vi "Get Rx and Tx Status Channels for Message.vi"(8 "error in":errorcluster, 11 "message refs":T1[](array[typedef]) format="%.0x") -> (0 "error out":errorcluster, 1 "Rx status channels":T1[](array[typedef]) format="%.0x", 2 "Tx status channels":T1[](array[typedef]) format="%.0x", 3 "message refs":T1[](array[typedef]) format="%.0x")   [LabVIEW 2023, in "Ballard MIL-STD-1553 Scripting.lvlib"]
uses:
  Ballard MIL-STD-1553 Scripting.lvlib
  <vilib>/NI VeriStand/Custom Device API/Custom Device Item Ref.ctl
  Shared/Direction.ctl
  Constants.vi
  <vilib>/NI VeriStand/Custom Device API/Custom Device API.lvlib
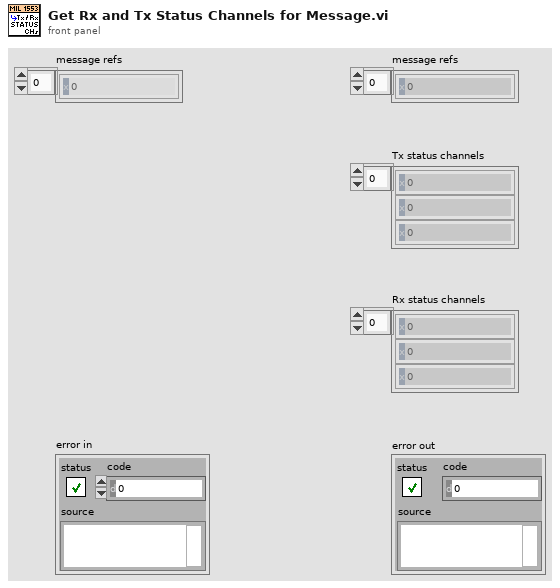
[diagram p1: front panel]
types:
  T1 = typedef "Custom Device API.lvlib/Custom Device Item Ref.ctl" = u64
  T2 = typedef "Direction.ctl" = enum16{"Rx", "Tx"}
  T3 = typedef "Message Type.ctl" = string
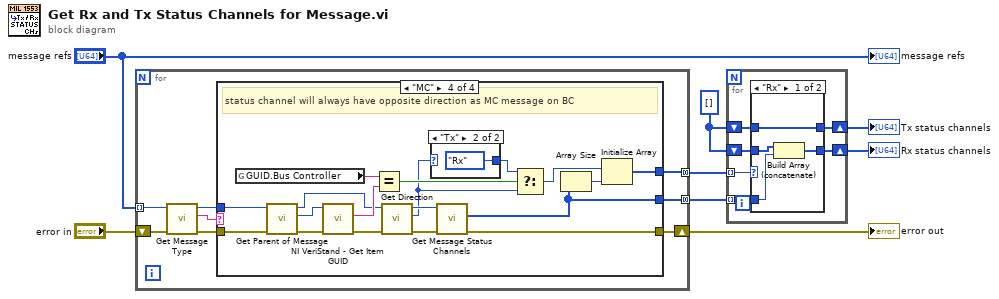
[diagram p0: block diagram]
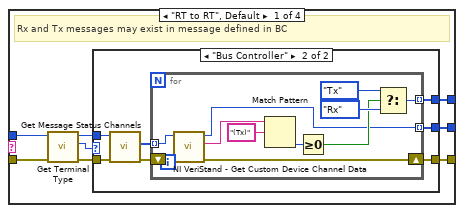
[diagram p2: hidden frame]
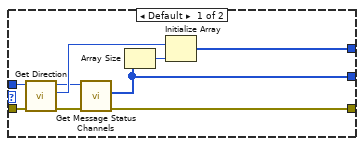
[diagram p3: hidden frame]
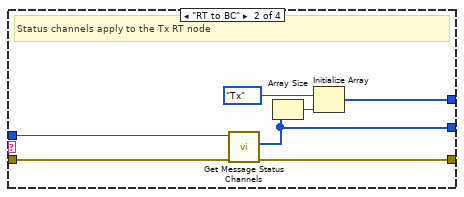
[diagram p4: hidden frame]
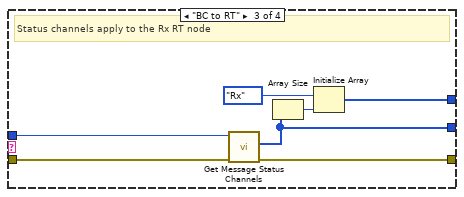
[diagram p5: hidden frame]
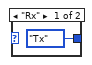
[diagram p6: hidden frame]
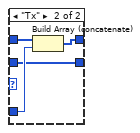
[diagram p7: hidden frame]
diagram:
  w6 = T1[] [] ("Rx status channels")
  n1 = for {
    tunnel: [w10] -> w3 mode=concatenating
    shift-right: [w11] -> w1
    shift-left: "error in" -> [w15]
    tunnel: "message refs" -> [w16] mode=indexing
    tunnel: [w9] -> w2 mode=concatenating
    n2 = call "Get Message Type.vi"("error in"=w15, "message in"=w16) -> ("error out"=w13:errorcluster, "message type"=w14:T3, "message out"=w12:T1)  [unwired: 6 in, 1 out]
    n3 = case shown="\"MC\"" w14 {
      tunnel: w13 -> [w20 w52 w59 w69]
      tunnel: w12 -> [w21 w53 w60 w70]
      tunnel: [w22 w58 w65 w81] -> w11
      tunnel: [w23 w55 w62 w82] -> w10
      tunnel: [w24 w54 w61 w83] -> w9
      frame "RT to RT", Default {
        # "Rx and Tx messages may exist in message defined in BC"
        n4 = call "Get Terminal Type.vi"("error in"=w20, "message in"=w21) -> ("error out"=w19:errorcluster, "terminal type"=w17:enum16{"Bus Controller", "Remote Terminal"}, "message out"=w18:T1)  [unwired: 7 in]
        n5 = case shown="\"Bus Controller\"" w17 {
          tunnel: w18 -> [w33 w40]
          tunnel: w19 -> [w32 w39]
          tunnel: [w30 w36] -> w24
          tunnel: [w26 w35] -> w23
          tunnel: [w25 w34] -> w22
          frame Default {
            n6 = call "Get Direction.vi"("error in"=w32, "message in"=w33) -> ("error out"=w27:errorcluster, "direction"=w29:T2, "message out"=w28:T1)  [unwired: 6 in, 1 out]
            n7 = call "Get Message Status Channels.vi"("error in"=w27, "message in"=w28) -> ("error out"=w25:errorcluster, "status channels"=w26:T1[])  [unwired: 6 in, 2 out]
            n8 = Array Size(array=w26) -> (size(s)=w31:i32)
            n9 = Initialize Array(w29, w31) -> (w30:T2[])
          }
          frame "Bus Controller" {
            n10 = call "Get Message Status Channels.vi"("error in"=w39, "message in"=w40) -> ("error out"=w38:errorcluster, "status channels"=w37:T1[])  [unwired: 6 in, 2 out]
            n11 = for {
              tunnel: w37 -> [w48] mode=indexing
              tunnel: [w44] -> w36 mode=indexing
              tunnel: [w41] -> w35 mode=indexing
              shift-right: [w43] -> w34
              shift-left: w38 -> [w49]
              n12 = call <vilib>:"NI VeriStand - Get Custom Device Channel Data.vi"("error in (no error)"=w49, "Channel Ref in"=w48) -> ("error out"=w43:errorcluster, "Channel Name"=w51:string, "Channel Ref out"=w41:T1)  [unwired: 4 in, 3 out]
              n13 = Match Pattern(string=w51, regular expression="(Tx)") -> (offset past match=w47:i32)  [unwired: 1 in, 3 out]
              n14 = Greater Or Equal To 0?(x=w47) -> (x >= 0?=w42:bool)
              n15 = Select(t=Direction."Tx" ("direction"), s=w42, f=Direction."Rx" ("direction")) -> (s? t:f=w44:T2)
            }
          }
        }
      }
      frame "RT to BC" {
        # "Status channels apply to the Tx RT node"
        n16 = call "Get Message Status Channels.vi"("error in"=w52, "message in"=w53) -> ("error out"=w58:errorcluster, "status channels"=w55:T1[])  [unwired: 6 in, 2 out]
        n17 = Array Size(array=w55) -> (size(s)=w56:i32)
        n18 = Initialize Array(Direction."Tx" ("direction"), w56) -> (w54:T2[])
      }
      frame "BC to RT" {
        # "Status channels apply to the Rx RT node"
        n19 = call "Get Message Status Channels.vi"("error in"=w59, "message in"=w60) -> ("error out"=w65:errorcluster, "status channels"=w62:T1[])  [unwired: 6 in, 2 out]
        n20 = Array Size(array=w62) -> (size(s)=w63:i32)
        n21 = Initialize Array(Direction."Rx" ("direction"), w63) -> (w61:T2[])
      }
      frame "MC" {
        # "status channel will always have opposite direction as MC message on BC"
        n22 = global read "Constants.vi" "GUID.Bus Controller"() -> (w76:string)
        n23 = call "Get Parent of Message.vi"("error in"=w69, "message"=w70) -> ("error out"=w68:errorcluster, "parent of message"=w67:T1, "message out"=w66:T1)  [unwired: 7 in]
        n24 = call <vilib>:"NI VeriStand - Get Item GUID.vi"("error in (no error)"=w68, "Item Ref in"=w67) -> ("error out"=w75:errorcluster, "GUID"=w77:string)  [unwired: 7 in, 1 out]
        n25 = Equal?(x=w76, y=w77) -> (x = y?=w74:bool)
        n26 = call "Get Direction.vi"("error in"=w75, "message in"=w66) -> ("error out"=w78:errorcluster, "direction"=w72:T2, "message out"=w79:T1)  [unwired: 6 in, 1 out]
        n27 = case shown="\"Tx\"" w72 {
          tunnel: [Direction."Tx" ("direction") Direction."Rx" ("direction")] -> w71
          frame "Rx" {
          }
          frame "Tx" {
          }
        }
        n28 = call "Get Message Status Channels.vi"("error in"=w78, "message in"=w79) -> ("error out"=w81:errorcluster, "status channels"=w82:T1[])  [unwired: 6 in, 2 out]
        n29 = Select(t=w71, s=w74, f=w72) -> (s? t:f=w73:T2)
        n30 = Array Size(array=w82) -> (size(s)=w80:i32)
        n31 = Initialize Array(w73, w80) -> (w83:T2[])
      }
    }
  }
  "error out" <- w1
  n32 = for {
    tunnel: w3 -> [w91] mode=indexing
    shift-right: [w87] -> w5
    shift-left: w6 -> [w90]
    shift-right: [w88] -> w4
    shift-left: w6 -> [w89]
    tunnel: w2 -> [w86] mode=indexing
    n33 = case shown="\"Rx\"" w86 {
      tunnel: w91 -> [w93 w98]
      tunnel: w90 -> [w92 w99]
      tunnel: w89 -> [w95 w97]
      tunnel: [w94 w97] -> w88
      tunnel: [w92 w96] -> w87
      frame "Rx" {
        n34 = Build Array (concatenate)(w95, w93) -> (w94:T1[])
      }
      frame "Tx" {
        n35 = Build Array (concatenate)(w99, w98) -> (w96:T1[])
      }
    }
  }
  "Tx status channels" <- w5
  "Rx status channels" <- w4
  "message refs" <- "message refs"
